vi "Get Clock State.vi"(0 "handshake in":refnum<k21>) -> (4 "clock valid":bool)   [LabVIEW 2019]
uses:
  <vilib>/rvi/DataTransferAndStorage/Container/Common/niFpgaContainerExecOnDevCompGetState.vi
  <vilib>/rvi/Emulation/niFpgaEmulationIsFPGAContextNoSignature.vi
  <vilib>/rvi/DataTransferAndStorage/Container/Common/niFpgaContainerGetUniqueNameForEmu.vi
  <vilib>/rvi/eio/common/nirviEmuReportErrorAndStop.vi
  <vilib>/rvi/Emulation/niFpgaSctlEmulationGetInTimedLoop.vi
  <vilib>/rvi/Emulation/niFpgaProcessEmulError.vi
  <vilib>/rvi/DataTransferAndStorage/Container/XNode/niFpgaContainer.xnode
  <vilib>/rvi/DataTransferAndStorage/Handshake/Emulation/niFpgaHandshakeEmulationRefIn.vi
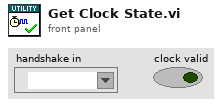
[diagram p1: front panel]
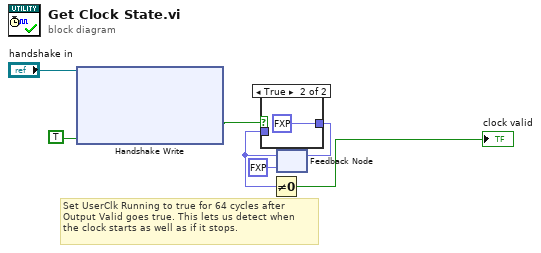
[diagram p0: block diagram]
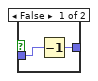
[diagram p2: hidden frame]
diagram:
  # "Set UserClk Running to true for 64 cycles after\nOutput Valid goes true. This lets us detect when \nthe clock starts as well as if it stops."
  n1 = xnode ("Handshake Write")("Ready for Output"=TRUE, "Handshake In"="handshake in") -> ("Output Valid"=w7:bool)  [unwired: 2 out]
  n2 = feedback #1(fxp<+,6,6> 0.0) -> (w2:fxp<+,6,6>)
  n3 = case shown="True" w7 {
    tunnel: [w8 fxp<+,6,6> 63.0] -> w1
    tunnel: w2 -> [w9 _]
    frame False {
      n4 = Decrement(x=w9) -> (x-1=w8:fxp<+,6,6>)
    }
    frame True {
    }
  }
  n5 = Not Equal To 0?(x=w2) -> (x != 0?=→"clock valid":bool)
  n6 = feedback-in #1(w1) -> ()
